vi "Stop Core.vi"(10 "final error code":i32, 11 "Nested in":refnum<class "Nested.lvclass">) -> (3 "Nested out":refnum<class "Nested.lvclass">)   [LabVIEW 2020, in "Nested.lvlib" / "Nested.lvclass"]
doc: "(<B>Filename</B>: Actor Framework.lvlib:Actor.lvclass:Stop Core.vi)\n\nDefines what the actor does before it stops. Use the <B>final error code</B> input to determine whether the actor shut down in response to an error.\n\nBy default, this method passes the Stop message along to all auto-stop nested actors. A descendant class may override this method to define additional behavior, such as shutting down any processes the actor initiated in its override of the Actor Core method."
uses:
  Nested.lvclass
  Nested.lvclass/Nested.ctl
  <vilib>/ActorFramework/Actor/Actor.lvclass
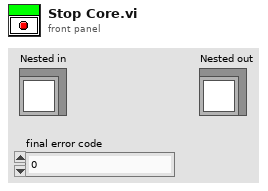
[diagram p1: front panel]
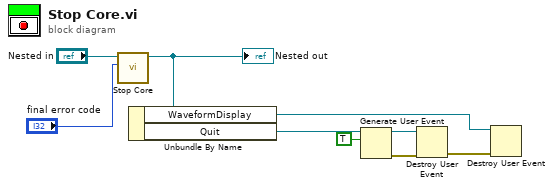
[diagram p0: block diagram]
diagram:
  n1 = call-parent "Stop Core.vi"("final error code"="final error code", "Actor in"="Nested in") -> ("Actor out"=w7:refnum<class "Nested.lvclass">)  [unwired: 9 in]
  "Nested out" <- w7
  n2 = Unbundle By Name(w7) -> ("WaveformDisplay"=w1:refnum<user-event>, "Quit"=w6:refnum<user-event>)
  n3 = Generate User Event(user event=w6, event data cluster=TRUE ("event data")) -> (user event out=w5:refnum<user-event>, error out=w4:errorcluster)  [unwired: 2 in]
  n4 = Destroy User Event(user event=w5, error in=w4) -> (error out=w2:errorcluster)
  n5 = Destroy User Event(user event=w1, error in=w2) -> ()  [unwired: 1 out]
